vi "lab_3.vi"() -> ()   [LabVIEW 2016]
uses:
  <vilib>/myRIO/Instrument Drivers/Onboard Devices/Accelerometer/typedefs/Accelerometer Reference.ctl
  <vilib>/myRIO/Common/Instrument Driver Framework/Utilities/typedefs/myRIO Generic Hardware Reference.ctl
  <vilib>/myRIO/Common/Instrument Driver Framework/Utilities/typedefs/Hardware Version Enum.ctl
  <vilib>/myRIO/Common/Instrument Driver Framework/Utilities/typedefs/myRIO v1.0 Reference.ctl
  <vilib>/myRIO/Common/Instrument Driver Framework/Utilities/typedefs/Generic FPGA Reference.ctl
  <vilib>/myRIO/Common/Instrument Driver Framework/myRIO v1.0/Accelerometer/typedefs/Accelerometer Channels List.ctl
  <vilib>/myRIO/Common/Instrument Driver Framework/myRIO v1.0/Accelerometer/typedefs/Accelerometer Channels Enum.ctl
  <vilib>/userdefined/High Color/nirio_resource_hc.ctl
  <vilib>/myRIO/Instrument Drivers/Onboard IO/DIO/typedefs/DIO Reference.ctl
  <vilib>/myRIO/Common/Instrument Driver Framework/myRIO v1.0/DIO/typedefs/DIO Channels List.ctl
  <vilib>/myRIO/Common/Instrument Driver Framework/myRIO v1.0/DIO/typedefs/DIO Channels Enum.ctl
  <vilib>/myRIO/Common/Instrument Driver Framework/Utilities/vis/Is FPGA Ref Available.vi
  <vilib>/myRIO/Common/Instrument Driver Framework/myRIO v1.0/Accelerometer/vis/myRIO v1.1 Open Accelerometer.vi
  <vilib>/myRIO/Instrument Drivers/Onboard Devices/Accelerometer/vis/Read.vi
  <vilib>/myRIO/Common/Instrument Driver Framework/myRIO v1.0/DIO/vis/myRIO v1.1 Open DIO.vi
  <vilib>/myRIO/Instrument Drivers/Onboard IO/DIO/vis/Write.vi
  <vilib>/myRIO/Common/Instrument Driver Framework/Utilities/vis/Validate Channels.vi
  <vilib>/myRIO/Common/Instrument Driver Framework/myRIO v1.0/Accelerometer/vis/myRIO v1.0 Reserve Accelerometer.vi
  <vilib>/myRIO/Common/Instrument Driver Framework/myRIO v1.0/UART/vis/myRIO v1.0 Close UART.vi
  <vilib>/myRIO/Common/Instrument Driver Framework/myRIO v1.0/DIO/vis/myRIO v1.0 Reserve DIO.vi
  <vilib>/myRIO/Common/Instrument Driver Framework/myRIO v1.0/Resource Manager/vis/myRIO v1.0 Reserve Channel List.vi
  <vilib>/myRIO/Common/Instrument Driver Framework/myRIO v1.0/Accelerometer/vis/myRIO v1.0 Build MUX Configuration Accelerometer.vi
  <vilib>/myRIO/Common/Instrument Driver Framework/myRIO v1.0/DIO/vis/myRIO v1.0 Build MUX Configuration DIO.vi
  <vilib>/myRIO/Common/Instrument Driver Framework/myRIO v1.0/Resource Manager/vis/myRIO v1.0 Reserve Channel.vi
  <vilib>/myRIO/Common/Instrument Driver Framework/myRIO v1.0/Resource Manager/vis/myRIO v1.0 Unreserve Channel.vi
  <vilib>/myRIO/Common/Instrument Driver Framework/myRIO v1.0/Resource Manager/vis/myRIO v1.0 Create Configuration List.vi
  <vilib>/myRIO/Common/Instrument Driver Framework/myRIO v1.0/Resource Manager/vis/myRIO v1.0 Build Mutex Name.vi
  <vilib>/Utility/VariantDataType/GetNumericInfo.vi
  <vilib>/Utility/error.llb/Error Cluster From Error Code.vi
  <vilib>/myRIO/Common/Instrument Driver Framework/myRIO v1.0/myRIO v1.1 Open.vi
  <vilib>/myRIO/Common/Instrument Driver Framework/myRIO v1.0/Accelerometer/vis/myRIO v1.0 Get Scaling Constant Accelerometer.vi
  <vilib>/myRIO/Common/Instrument Driver Framework/Utilities/vis/IO Manager.vi
  <vilib>/myRIO/Common/Instrument Driver Framework/Utilities/vis/Configuration Manager.vi
  <vilib>/myRIO/Common/Instrument Driver Framework/myRIO v1.0/myRIO v1.0 Close.vi
  <vilib>/myRIO/Common/Instrument Driver Framework/myRIO v1.0/Accelerometer/vis/myRIO v1.0 Read Accelerometer.vi
  <vilib>/Analysis/Matrix/Numeric/Conversions/Matrix To Array - RM.vi
  <vilib>/myRIO/Common/Instrument Driver Framework/Utilities/vis/FPGA Ref Manager.vi
  <vilib>/myRIO/Common/Instrument Driver Framework/myRIO v1.0/myRIO v1.0 Reset FPGA.vi
  <vilib>/myRIO/Common/Instrument Driver Framework/myRIO v1.0/IRQ/vis/myRIO v1.0 IRQ Info FGV.vi
  <vilib>/myRIO/Common/Instrument Driver Framework/myRIO v1.0/IRQ/vis/myRIO v1.0 Timer IRQ Info FGV.vi
  <vilib>/myRIO/Common/Instrument Driver Framework/myRIO v1.0/IRQ/vis/myRIO v1.0 ISR Agent.vi
  <vilib>/myRIO/Common/Instrument Driver Framework/myRIO v1.0/Resource Manager/vis/myRIO v1.0 Configure IO.vi
  <vilib>/myRIO/Common/Instrument Driver Framework/myRIO v1.0/DIO/vis/myRIO v1.0 Write DIO.vi
  <vilib>/myRIO/Express VI/Onboard Devices/Accelerometer/Accelerometer Express VI.xnode
  <vilib>/myRIO/Instrument Drivers/Onboard Devices/Accelerometer/vis/myRIO Accelerometer Open.xnode
  <vilib>/myRIO/Express VI/Onboard Devices/LED/LED Express VI.xnode
  <vilib>/myRIO/Instrument Drivers/Onboard IO/DIO/vis/myRIO DIO Open.xnode
  <vilib>/myRIO/Instrument Drivers/Onboard Devices/Accelerometer/Accelerometer.lvlib
  <vilib>/myRIO/Instrument Drivers/Utilities/Utilities.lvlib
  <vilib>/Analysis/Matrix/NI_Matrix.lvlib
  <vilib>/myRIO/Instrument Drivers/Onboard IO/DIO/DIO.lvlib
panel:
  in  "ACTIVATION":bool
  in  "STOP INFERENCE":bool
  in  "WRITE WEIGHTS":bool=TRUE
  in  "WRITE DATA":bool
  in  "Weights Source":bool=TRUE
  in  "START INFERENCE":bool
  in  "BEGIN TRAINING MODE":bool
  in  "BEGIN INFERENCE MODE":bool
  in  "Mode Initialize":T1(ring)=enum."inference"
  in  "Validation Split":dbl=0.20000000000000015 min=0.0 max=1.0 step=0.1
  out "Loss":cluster{dbl, dbl}(graph)
  in  "Learning Rate":dbl=0.01 step=0.005
  out "Training Status":string
  in  "START TRAINING":bool
  out "Input Data":dbl[][](array[numeric])
  out "Total # of Samples":i32
  out "Targets":dbl[](array[numeric])
  in  "STOP TRAINING":bool
  in  "# ouputs":i32=3
  in  "# inputs":i32=5
  in  "# nodes per hidden layer":i32=8
  in  "# hidden layers":i32=1
  in  "Data Source":bool=TRUE
  out "Shuffled Targets":dbl[](array[numeric])
  out "Shuffled Input Data":dbl[][](array[numeric])
  in  "# of Samples to collect":i32
  in  "NEXT TARGET":bool
  out "Mode Status":string
  in  "Set Target (0, 1, 2)":i8 min=0 max=3
  out "# of Samples for current target":i32
  in  "Main Loop STOP":bool
  out "error out":errorcluster
  out "MyRIO Accelerometer":T2(graph)
  out "MyRIO Angular Position":cluster{dbl, dbl}(graph)
  in  "FILTER ON/OFF":bool=TRUE
  in  "Smoothing Factor":dbl(slide)=0.17171717171717182 min=-1.0 max=1.0 step=0.05 scale=-1.0..1.0
  # "Lab 4: Example Submission"
  # "Author: Adam Cavatassi, McGill University, 2018"
  # "Main Control"
  # "Training Control"
  # "ON - Shared Variable"
  # "OFF - Local Data"
  # "Inference Control"
  # "ON - Shared Variable"
  # "OFF - Local Data"
  # "ON - reLU"
  # "OFF - sigmoid Data"
  # "Data Generation Control"
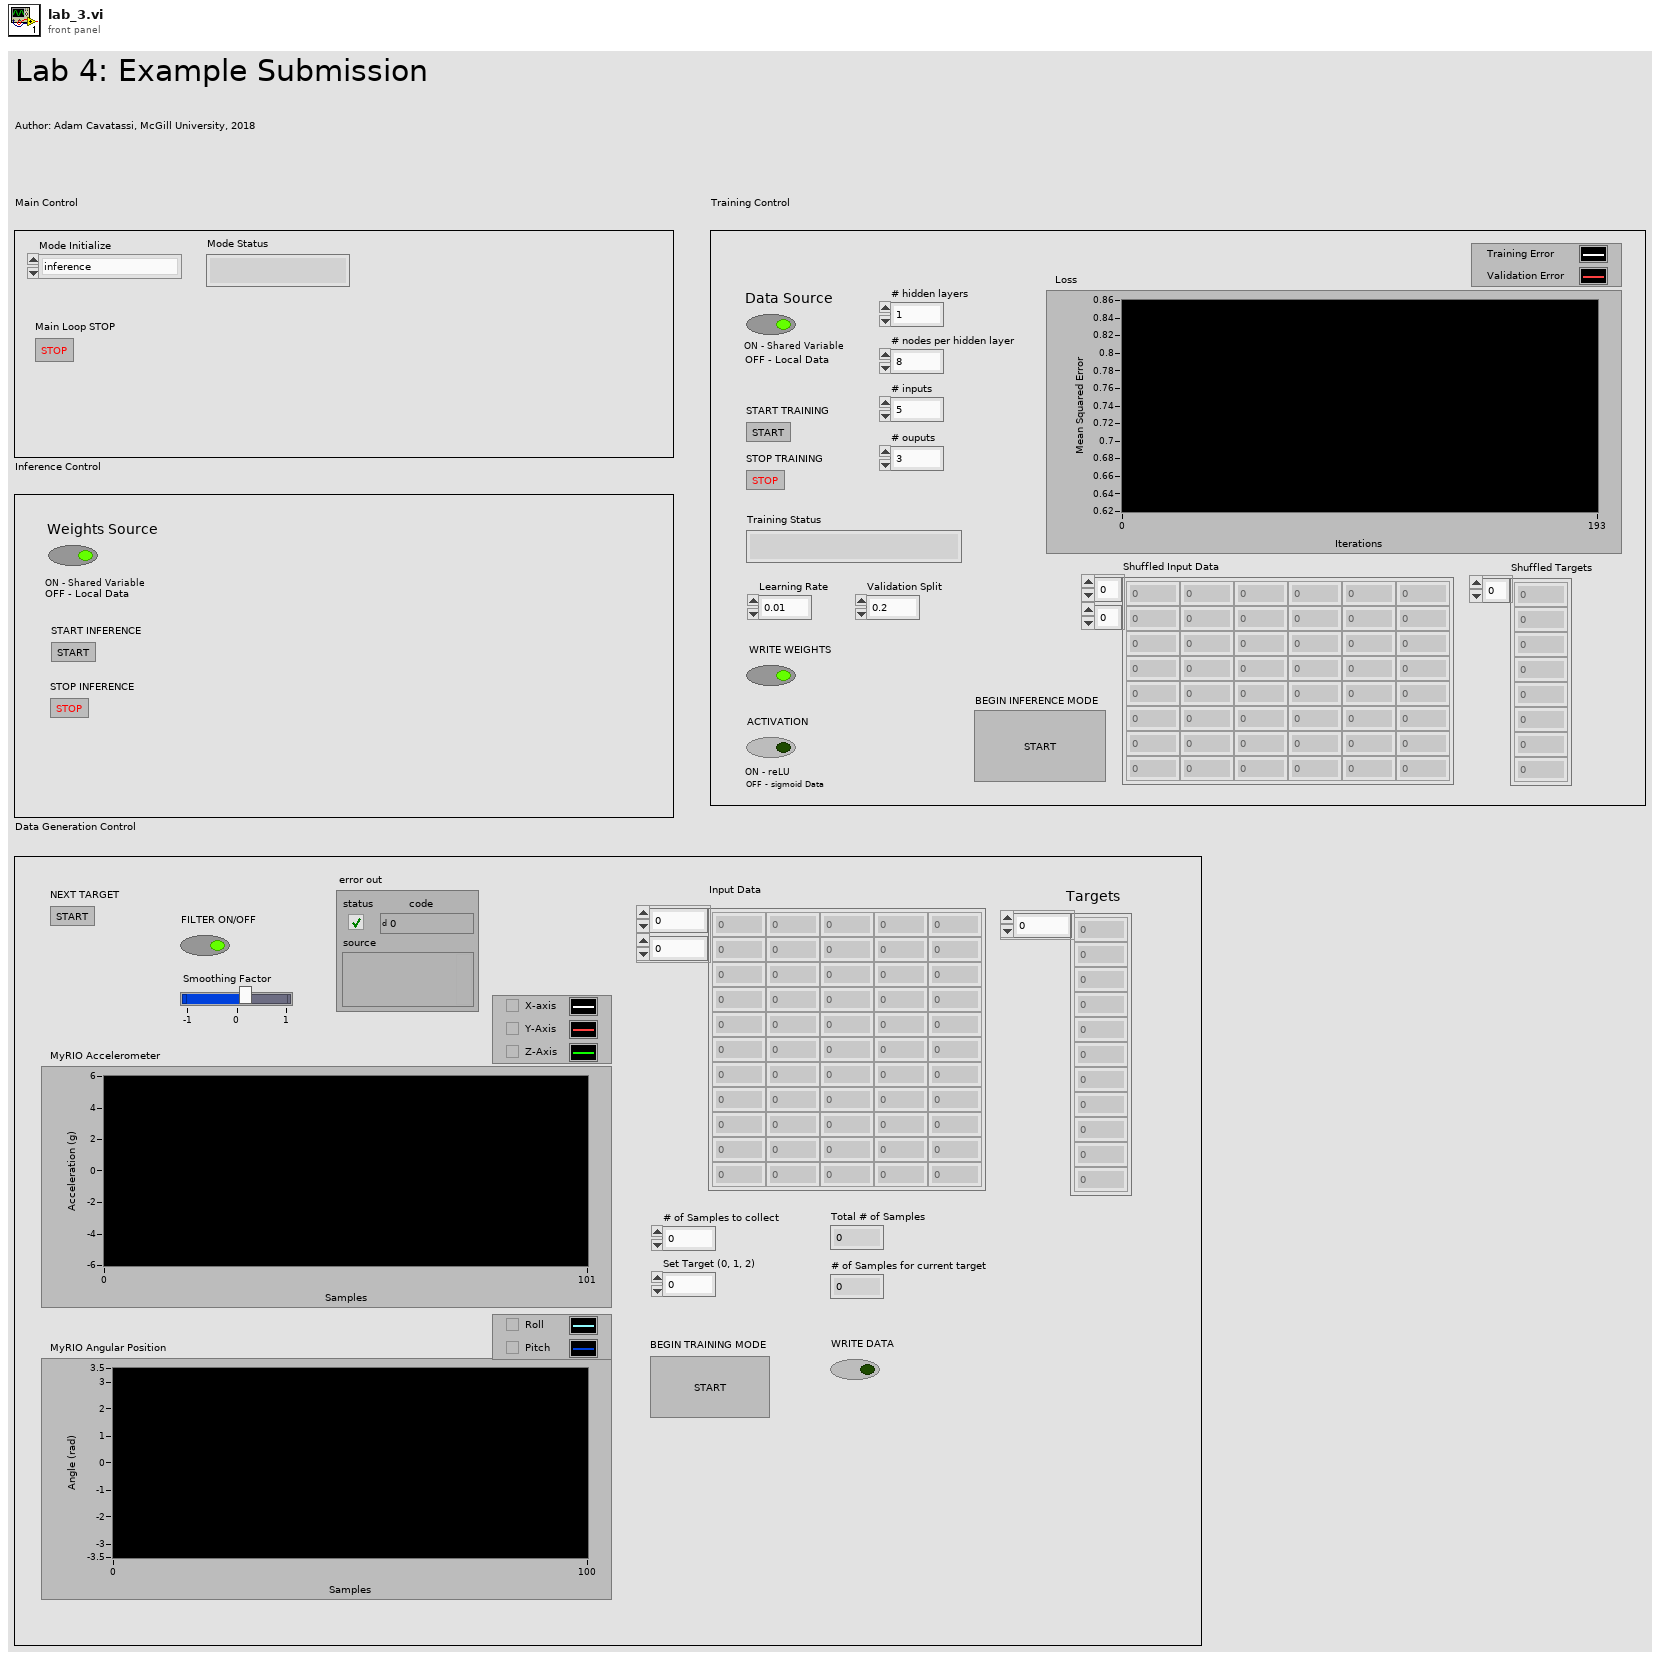
[diagram p1: front panel]
types:
  T1 = enum16{"data_collection", "network_train", "inference"}
  T2 = cluster{"X-Axis":dbl, "Y-Axis":dbl, "Z-Axis":dbl}
  T3 = typedef "Accelerometer.lvlib/Accelerometer Reference.ctl" = cluster{"myRIO Reference":T4, "Accelerometer Channels List":T8, "LSB Weight":dbl}
  T4 = typedef "myRIO Generic Hardware Reference.ctl" = cluster{"myRIO Model":T5, "myRIO Hardware Reference":T6}
  T5 = typedef "Hardware Version Enum.ctl" = enum16{"Unknown", "myRIO-1900", "myRIO-1950", "roboRIO", "NI ELVIS RIO CM"}
  T6 = typedef "myRIO v1.0 Reference.ctl" = cluster{"Generic FPGA Reference":T7, "Allow multiple opens":bool}
  T7 = typedef "Generic FPGA Reference.ctl" = refnum<k20>
  T8 = typedef "Accelerometer Channels List.ctl" = T9[]
  T9 = typedef "Accelerometer Channels Enum.ctl" = enum16{"Not Connected", "X-Axis", "Y-Axis", "Z-Axis"}
  T10 = typedef "nirio_resource_hc.ctl" = tag
  T11 = typedef "DIO.lvlib/DIO Reference.ctl" = cluster{"myRIO Reference":T4, "DIO Channels List":T12}
  T12 = typedef "DIO Channels List.ctl" = T13[]
  T13 = typedef "DIO Channels Enum.ctl" = enum16{"Not Connected", "C/DIO0", "C/DIO1", "C/DIO2", "C/DIO3", "C/DIO4", "C/DIO5", "C/DIO6", "C/DIO7", "A/DIO0", "A/DIO1", "A/DIO2", "A/DIO3", "A/DIO4", "A/DIO5", "A/DIO6", "A/DIO7", "A/DIO8", "A/DIO9", "A/DIO10", "A/DIO11", "A/DIO12", "A/DIO13", "A/DIO14", "A/DIO15", "B/DIO0", "B/DIO1", "B/DIO2", "B/DIO3", "B/DIO4", "B/DIO5", "B/DIO6", "B/DIO7", "B/DIO8", "B/DIO9", "B/DIO10", "B/DIO11", "B/DIO12", "B/DIO13", "B/DIO14", "B/DIO15", "LED0", "LED1", "LED2", "LED3", "Button0", "DIO/DIO0", "DIO/DIO1", "DIO/DIO2", "DIO/DIO3", "DIO/DIO4", "DIO/DIO5", "DIO/DIO6", "DIO/DIO7", "DIO/DIO8", "DIO/DIO9", "SPI/CS0", "SPI/CS1", "SPI/CS2", "SPI/CS3", "LED RADIO (Green)", "LED RADIO (Red)", "LED COMM (Green)", "LED COMM (Red)", "LED MODE (Green)", "LED MODE (Red)"}
  T14 = typedef "NI_Matrix.lvlib/RealMatrix.ctl" = dbl[][]
  T15 = cluster{"number: 0 to 1":dbl, dbl[], "Numeric":dbl}
  T16 = cluster{"number: 0 to 1":dbl, dbl[], "Numeric":dbl}[]
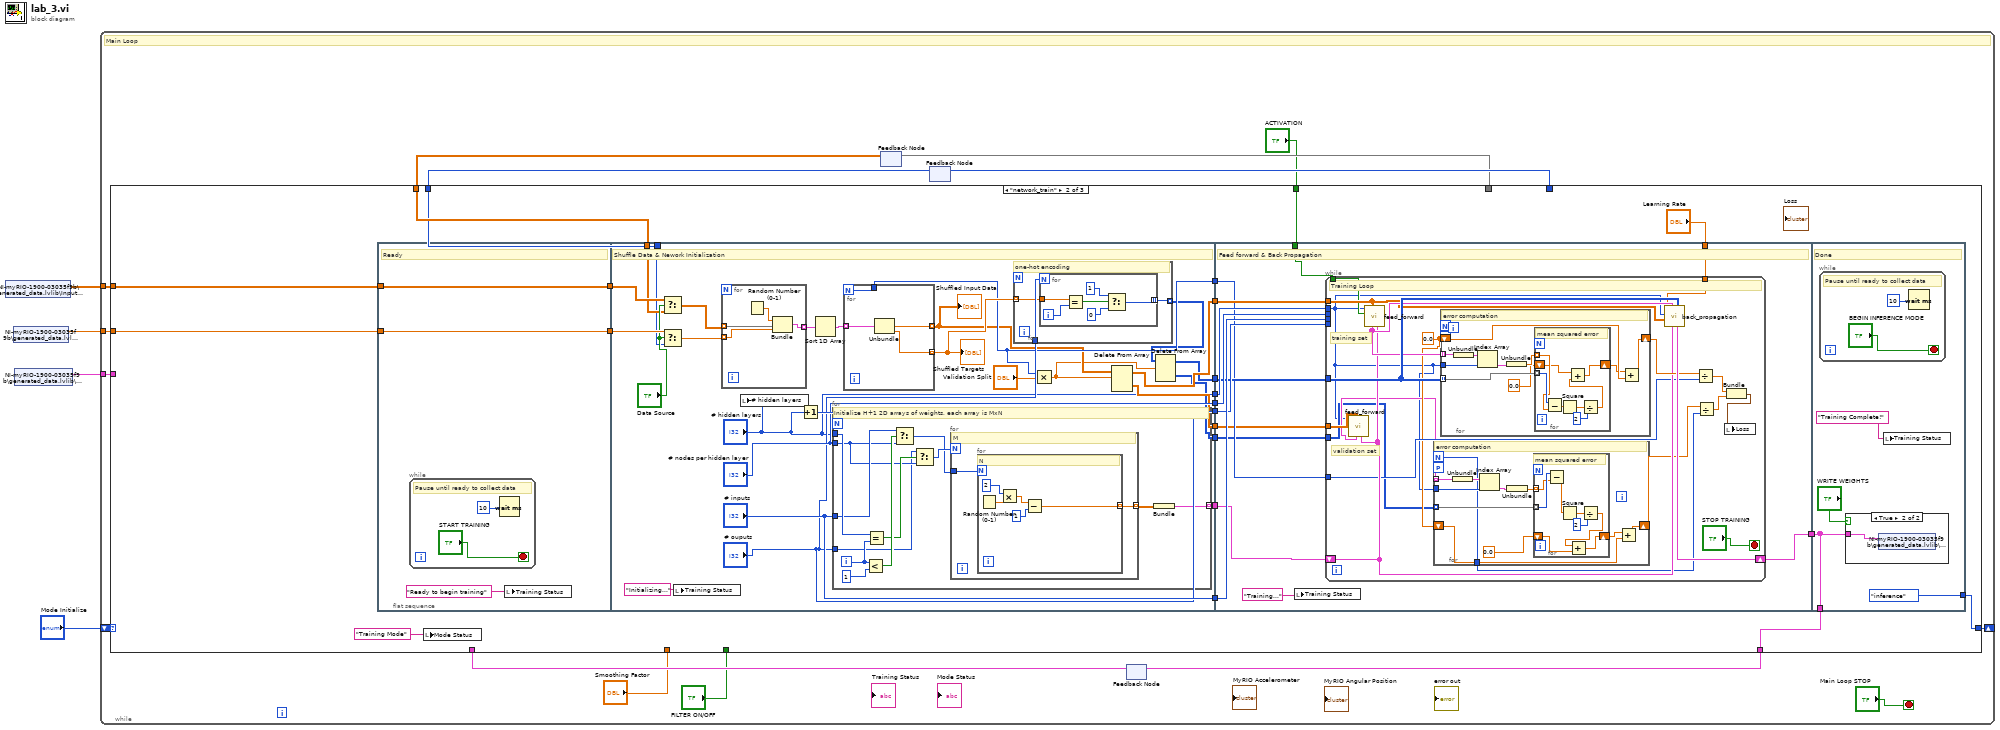
[diagram p0: block diagram]
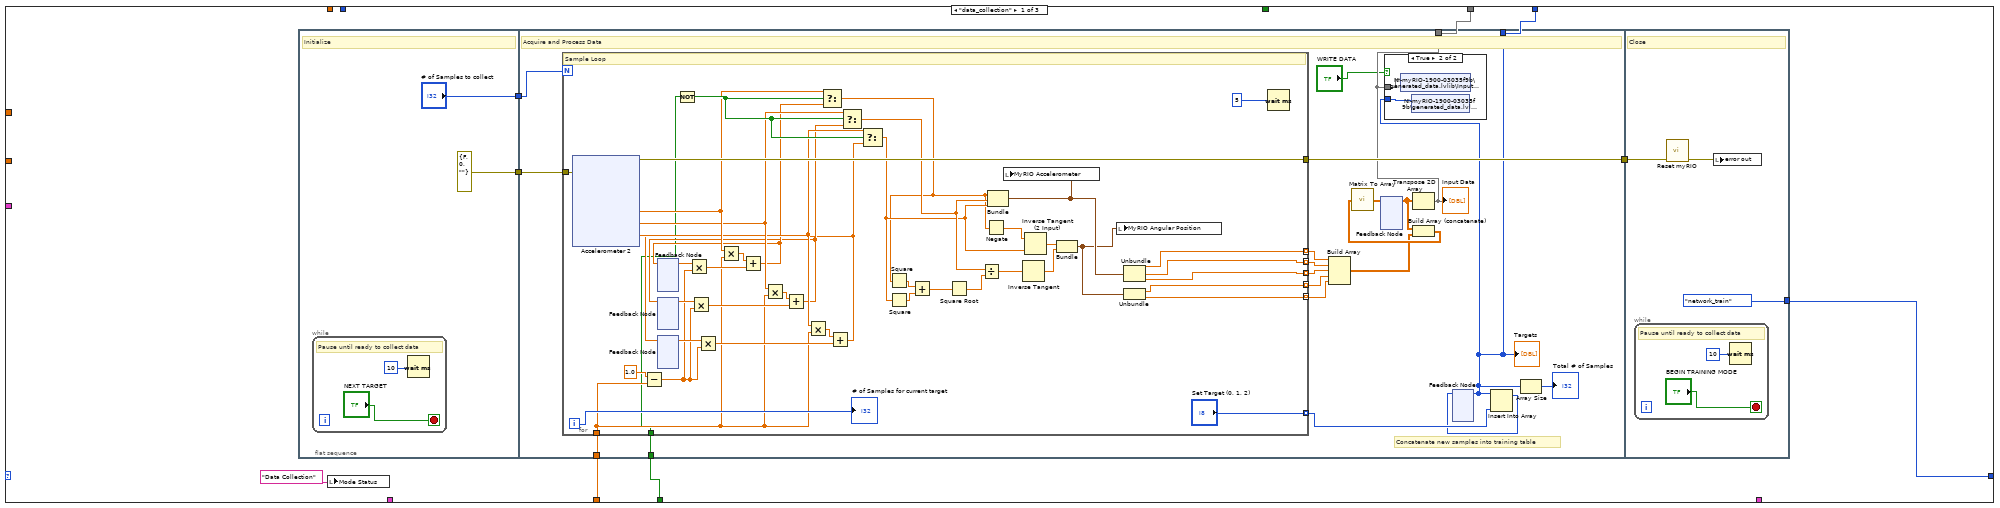
[diagram p2: hidden frame]
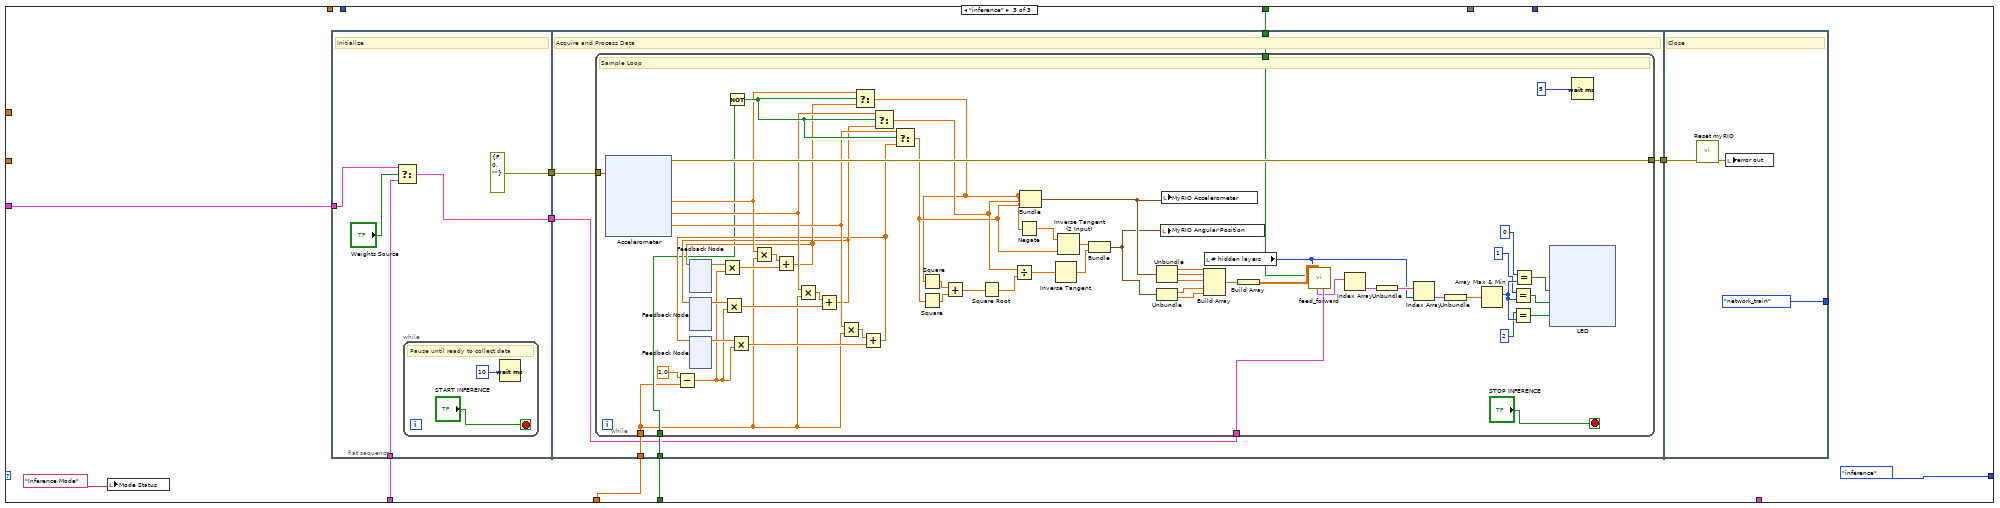
[diagram p5: hidden frame]
diagram:
  n1 = shared-variable "NI-myRIO-1900-03035f9b\\generated_data.lvlib\\Input Data"() -> (w3:dbl[][])  [unwired: 1 in, 1 out]
  n2 = shared-variable "NI-myRIO-1900-03035f9b\\generated_data.lvlib\\Targets"() -> (w4:dbl[])  [unwired: 1 in, 1 out]
  n3 = shared-variable "NI-myRIO-1900-03035f9b\\generated_data.lvlib\\Weights"() -> (w1:cluster{dbl[][]}[])  [unwired: 1 in, 1 out]
  n4 = while {
    shift-right: [w18] -> _
    shift-left: "Mode Initialize" -> [w19]
    tunnel: w3 -> [w17]
    tunnel: w4 -> [w16]
    tunnel: w1 -> [w10]
    stop <- "Main Loop STOP" stop-if-true
    # "Main Loop"
    n5 = feedback #1() -> (w12:dbl[][])  [unwired: 1 in]
    n6 = feedback #2() -> (w14:i8[])  [unwired: 1 in]
    n7 = feedback #3() -> (w8:cluster{dbl[][]}[])  [unwired: 1 in]
    n8 = case shown="\"network_train\"" w19 {
      tunnel: [w26 _ _] -> w13
      tunnel: [w25 _ _] -> w15
      tunnel: [w23 w147 T1."inference" ("NETWORK MODE")] -> w18
      tunnel: w17 -> [_ w163 _]
      tunnel: w16 -> [_ w162 _]
      tunnel: w12 -> [_ w161 _]
      tunnel: w14 -> [_ w160 _]
      tunnel: [_ w144 _] -> w9
      tunnel: w10 -> [_ _ w314]
      tunnel: w8 -> [_ _ w313]
      tunnel: "Smoothing Factor" -> [w21 _ w310]
      tunnel: "FILTER ON/OFF" -> [w20 _ w311]
      tunnel: "ACTIVATION" -> [_ w143 w309]
      frame "data_collection" {
        n9 = flat-sequence {
          tunnel: [errorcluster {"status"=FALSE, "code"=0, "source"=""} ("error in (no error)")] -> w28
          tunnel: ["# of Samples to collect"] -> w24
          tunnel: w28 -> [w52]
          tunnel: [w51] -> w27
          tunnel: [w37] -> w26
          tunnel: [w36] -> w25
          tunnel: w24 -> [w45]
          tunnel: w21 -> [w34]
          tunnel: w20 -> [w33]
          tunnel: w27 -> [w139]
          tunnel: [T1."network_train" ("NETWORK MODE")] -> w23
          frame #0 {
            # "Initialize"
            n10 = while {
              stop <- "NEXT TARGET" stop-if-true
              # "Pause until ready to collect data"
              n11 = Wait (ms)(milliseconds to wait=10) -> ()  [unwired: 1 out]
            }
          }
          frame #1 {
            # "Concatenate new samples into training table"
            # "Acquire and Process Data"
            n12 = for {
              N: w45 -> [_]
              tunnel: w52 -> [w96]
              tunnel: [w95] -> w51
              tunnel: [w66] -> w46 mode=indexing
              tunnel: [w65] -> w50 mode=indexing
              tunnel: [w64] -> w49 mode=indexing
              tunnel: [w63] -> w48 mode=indexing
              tunnel: [w62] -> w47 mode=indexing
              tunnel: ["Set Target (0, 1, 2)"] -> w43 mode=indexing
              tunnel: w34 -> [w58]
              tunnel: w33 -> [w57]
              i -> [w59]
              # "Sample Loop"
              n13 = xnode "Accelerometer 2"("error in (no error)"=w96) -> ("X-Axis"=w75:dbl, "Y-Axis"=w74:dbl, "Z-Axis"=w71:dbl, "error out"=w95:errorcluster)
              n14 = Subtract(x=1.0, y=w58) -> (x-y=w76:dbl)
              n15 = feedback #4() -> (w86:dbl)  [unwired: 1 in]
              n16 = feedback #5() -> (w85:dbl)  [unwired: 1 in]
              n17 = feedback #6() -> (w84:dbl)  [unwired: 1 in]
              n18 = Not(x=w57) -> (.not. x?=w80:bool)
              n19 = Multiply(x=w86, y=w76) -> (x*y=w79:dbl)
              n20 = Multiply(x=w85, y=w76) -> (x*y=w78:dbl)
              n21 = Multiply(x=w84, y=w76) -> (x*y=w77:dbl)
              n22 = Multiply(x=w75, y=w58) -> (x*y=w72:dbl)
              n23 = Add(x=w72, y=w79) -> (x+y=w69:dbl)
              n24 = feedback-in #4(w69) -> ()
              n25 = Multiply(x=w74, y=w58) -> (x*y=w73:dbl)
              n26 = Add(x=w73, y=w78) -> (x+y=w68:dbl)
              n27 = feedback-in #5(w68) -> ()
              n28 = Multiply(x=w71, y=w58) -> (x*y=w70:dbl)
              n29 = Select(t=w75, s=w80, f=w69) -> (s? t:f=w61:dbl)
              n30 = Add(x=w70, y=w77) -> (x+y=w67:dbl)
              n31 = feedback-in #6(w67) -> ()
              n32 = Select(t=w74, s=w80, f=w68) -> (s? t:f=w82:dbl)
              n33 = Select(t=w71, s=w80, f=w67) -> (s? t:f=w81:dbl)
              n34 = Square(x=w61) -> (x^2=w89:dbl)
              n35 = Square(x=w81) -> (x^2=w94:dbl)
              n36 = Add(x=w89, y=w94) -> (x+y=w93:dbl)
              n37 = Square Root(x=w93) -> (sqrt(x)=w92:dbl)
              n38 = Divide(x=w82, y=w92) -> (x/y=w91:dbl)
              n39 = Negate(x=w61) -> (-x=w88:dbl)
              n40 = Bundle("X-Axis"=w61, "Y-Axis"=w82, "Z-Axis"=w81) -> (w56:T2)  [unwired: 1 in]
              n41 = local write "MyRIO Accelerometer"(w56) -> ()
              n42 = Inverse Tangent(1:w91) -> (0:w90:dbl)
              n43 = Inverse Tangent (2 Input)(1:w81, 2:w88) -> (0:w87:dbl)
              n44 = Bundle(w87, w90) -> (w55:cluster{dbl, dbl})  [unwired: 1 in]
              n45 = local write "MyRIO Angular Position"(w55) -> ()
              n46 = Unbundle(w56) -> ("X-Axis"=w66:dbl, "Y-Axis"=w65:dbl, "Z-Axis"=w64:dbl)
              n47 = Unbundle(w55) -> (w63:dbl, w62:dbl)
              n48 = Wait (ms)(milliseconds to wait=5) -> ()  [unwired: 1 out]
              "# of Samples for current target" <- w59
            }
            n49 = Build Array(w46, w50, w49, w48, w47) -> (w38:dbl[][])
            n50 = feedback #7() -> (w39:dbl[][])  [unwired: 1 in]
            n51 = Transpose 2D Array(2D array=w39) -> (transposed array=w37:dbl[][])
            "Input Data" <- w37
            n52 = Build Array (concatenate)(w39, w38) -> (w40:T14)
            n53 = call-poly <vilib>:"Matrix To Array.vi"("Real Matrix"=w40) -> ("Real 2D Array"=w41:dbl[][])
            n54 = feedback-in #7(w41) -> ()
            n55 = feedback #8() -> (w36:i8[])  [unwired: 1 in]
            "Targets" <- w36
            n56 = case shown="True" "WRITE DATA" {
              tunnel: w37 -> [_ w54]
              tunnel: w36 -> [_ w53]
              frame False {
              }
              frame True {
                n57 = shared-variable "NI-myRIO-1900-03035f9b\\generated_data.lvlib\\Input Data"(w54) -> ()  [unwired: 1 in, 1 out]
                n58 = shared-variable "NI-myRIO-1900-03035f9b\\generated_data.lvlib\\Targets"(w53) -> ()  [unwired: 1 in, 1 out]
              }
            }
            n59 = Insert Into Array(array=w36, new element=w43) -> (w42:i8[])  [unwired: 1 in]
            n60 = feedback-in #8(w42) -> ()
            n61 = Array Size(array=w36) -> (size(s)=→"Total # of Samples":i32)
          }
          frame #2 {
            # "Close"
            n62 = while {
              stop <- "BEGIN TRAINING MODE" stop-if-true
              # "Pause until ready to collect data"
              n63 = Wait (ms)(milliseconds to wait=10) -> ()  [unwired: 1 out]
            }
            n64 = call <vilib>:"Reset myRIO.vi"("error in (no error)"=w139) -> ("error out"=w137:errorcluster)  [unwired: 10 in]
            n65 = local write "error out"(w137) -> ()
          }
        }
        n66 = local write "Mode Status"("Data Collection") -> ()
      }
      frame "network_train" {
        n67 = flat-sequence {
          tunnel: w162 -> [w165]
          tunnel: w163 -> [w166]
          tunnel: [w166] -> w153
          tunnel: [w165] -> w152
          tunnel: w161 -> [w187]
          tunnel: w160 -> [w186]
          tunnel: [w182] -> w159
          tunnel: [w172] -> w158
          tunnel: ["# hidden layers"] -> w157
          tunnel: ["# nodes per hidden layer"] -> w156
          tunnel: ["# inputs"] -> w155
          tunnel: ["# ouputs"] -> w154
          tunnel: w153 -> [w192]
          tunnel: w152 -> [w190]
          tunnel: [w171] -> w151
          tunnel: [w177] -> w150
          tunnel: [w173] -> w149
          tunnel: [w170] -> w148
          tunnel: w159 -> [w238]
          tunnel: w158 -> [w244]
          tunnel: w157 -> [w243]
          tunnel: w156 -> [w242]
          tunnel: w155 -> [w241]
          tunnel: w154 -> [w240]
          tunnel: w151 -> [w237]
          tunnel: w150 -> [w236]
          tunnel: w149 -> [w235]
          tunnel: w148 -> [w234]
          tunnel: [w233] -> w145
          tunnel: w143 -> [w232]
          tunnel: "Learning Rate" -> [w231]
          tunnel: [T1."inference" ("NETWORK MODE")] -> w147
          tunnel: w145 -> [w304]
          tunnel: [w304] -> w144
          frame #0 {
            # "Ready"
            n68 = while {
              stop <- "START TRAINING" stop-if-true
              # "Pause until ready to collect data"
              n69 = Wait (ms)(milliseconds to wait=10) -> ()  [unwired: 1 out]
            }
            n70 = local write "Training Status"("Ready to begin training") -> ()
          }
          frame #1 {
            # "Shuffle Data & Nework Initialization"
            n71 = Select(t=w192, s="Data Source", f=w187) -> (s? t:f=w191:dbl[][])
            n72 = Select(t=w190, s="Data Source", f=w186) -> (s? t:f=w189:dbl[])
            n73 = local write "Training Status"("Initializing...") -> ()
            n74 = for {
              tunnel: w191 -> [w228] mode=indexing
              tunnel: w189 -> [w230] mode=indexing
              tunnel: [w227] -> w194 mode=indexing
              n75 = Random Number (0-1)() -> (number: 0 to 1=w229:dbl)
              n76 = Bundle("number: 0 to 1"=w229, w228, "Numeric"=w230) -> (w227:T15)  [unwired: 1 in]
            }
            n77 = local write "# hidden layers"("# hidden layers") -> ()
            n78 = Increment(x="# hidden layers") -> (x+1=w185:i32)
            n79 = Sort 1D Array(array=w194) -> (sorted array=w193:T16)
            n80 = for {
              N: w185 -> [_]
              tunnel: "# hidden layers" -> [w215]
              tunnel: "# inputs" -> [w214]
              tunnel: "# nodes per hidden layer" -> [w208]
              tunnel: "# ouputs" -> [w207]
              tunnel: [w204] -> w182 mode=indexing
              i -> [w209]
              # "Initialize H+1 2D arrays of weights, each array is MxN"
              n81 = Less?(x=w209, y=1) -> (x < y?=w213:bool)
              n82 = Equal?(x=w215, y=w209) -> (x = y?=w212:bool)
              n83 = Select(t=w214, s=w213, f=w208) -> (s? t:f=w206:i32)
              n84 = Select(t=w207, s=w212, f=w208) -> (s? t:f=w211:i32)
              n85 = for {
                N: w211 -> [_]
                tunnel: [w217] -> w205 mode=indexing
                tunnel: w206 -> [w216]
                # "M"
                n86 = for {
                  N: w216 -> [_]
                  tunnel: [w218] -> w217 mode=indexing
                  # "N"
                  n87 = Random Number (0-1)() -> (number: 0 to 1=w222:dbl)
                  n88 = Multiply(x=2, y=w222) -> (x*y=w220:dbl)
                  n89 = Subtract(x=w220, y=1) -> (x-y=w218:dbl)
                }
              }
              n90 = Bundle(w205) -> (w204:cluster{dbl[][]})  [unwired: 1 in]
            }
            n91 = for {
              N -> [w223]
              tunnel: w193 -> [w225] mode=indexing
              tunnel: [w226] -> w176 mode=indexing
              tunnel: [w224] -> w179 mode=indexing
              tunnel: [w223] -> w177
              n92 = Unbundle(w225) -> (w226:dbl[], "Numeric"=w224:dbl)  [unwired: 1 out]
            }
            "Shuffled Input Data" <- w176
            "Shuffled Targets" <- w179
            n93 = for {
              tunnel: "# ouputs" -> [w197]
              tunnel: w179 -> [w196] mode=indexing
              tunnel: [w195] -> w175 mode=indexing
              # "one-hot encoding"
              n94 = for {
                N: w197 -> [_]
                tunnel: w196 -> [w202]
                tunnel: [w198] -> w195 mode=indexing
                i -> [w203]
                n95 = Equal?(x=w202, y=w203) -> (x = y?=w201:bool)
                n96 = Select(t=1, s=w201, f=0) -> (s? t:f=w198:i32)
              }
            }
            n97 = Multiply(x=w177, y="Validation Split") -> (x*y=w174:dbl)
            n98 = Delete From Array(array=w176, length=w174) -> (deleted portion=w173:dbl[][], array with subset deleted=w172:dbl[][])  [unwired: 2 in]
            n99 = Delete From Array(array=w175, length=w174) -> (deleted portion=w170:i32[][], array with subset deleted=w171:i32[][])  [unwired: 2 in]
          }
          frame #2 {
            # "Feed forward & Back Propagation"
            n100 = local write "Training Status"("Training...") -> ()
            n101 = while {
              tunnel: w244 -> [w261]
              tunnel: w243 -> [w248]
              tunnel: w242 -> [_]
              tunnel: w241 -> [_]
              tunnel: w240 -> [_]
              shift-right: [w262] -> w233
              shift-left: w238 -> [w259]
              tunnel: w237 -> [w264]
              tunnel: w236 -> [w255]
              tunnel: w235 -> [w258]
              tunnel: w234 -> [w251]
              tunnel: w232 -> [w249]
              tunnel: w231 -> [w247]
              stop <- "STOP TRAINING" stop-if-true
              w253 = 0.0
              # "training set"
              # "validation set"
              # "Training Loop"
              n102 = call "feed_forward.vi"("Weights Cluster"=w259, "Input Data"=w258, "# hidden layers"=w248) -> ("Neurons"=w252:cluster{"Array":cluster{"Array 2":dbl[]}[]}[])  [unwired: 8 in]
              n103 = call "feed_forward.vi"("Weights Cluster"=w259, "Input Data"=w261, "act"=w249, "# hidden layers"=w248) -> ("Neurons"=w263:cluster{"Array":cluster{"Array 2":dbl[]}[]}[])  [unwired: 7 in]
              n104 = for {
                N -> [w265]
                tunnel: w248 -> [w273]
                tunnel: w252 -> [w275] mode=indexing
                shift-right: [w267] -> w254
                shift-left: w253 -> [w266]
                tunnel: w251 -> [w271] mode=indexing
                tunnel: [w265] -> w250
                workers-P: _ -> [_]
                # "error computation"
                n105 = Unbundle(w275) -> ("Array"=w274:cluster{"Array 2":dbl[]}[])
                n106 = Index Array(array=w274, index=w273) -> (element=w272:cluster{"Array 2":dbl[]})
                n107 = Unbundle(w272) -> ("Array 2"=w270:dbl[])
                n108 = for {
                  tunnel: w271 -> [w280] mode=indexing
                  tunnel: w270 -> [w276] mode=indexing
                  shift-right: [w278] -> w268
                  shift-left: 0.0 -> [w279]
                  # "mean squared error"
                  n109 = Subtract(x=w280, y=w276) -> (x-y=w283:dbl)
                  n110 = Square(x=w283) -> (x^2=w282:dbl)
                  n111 = Divide(x=w282, y=2) -> (x/y=w277:dbl)
                  n112 = Add(x=w277, y=w279) -> (x+y=w278:dbl)
                }
                n113 = Add(x=w268, y=w266) -> (x+y=w267:dbl)
              }
              n114 = for {
                tunnel: w264 -> [w293] mode=indexing
                tunnel: w263 -> [w292] mode=indexing
                tunnel: w248 -> [w285]
                shift-right: [w286] -> w260
                shift-left: w253 -> [w288]
                workers-P: _ -> [_]
                # "error computation"
                n115 = Unbundle(w292) -> ("Array"=w291:cluster{"Array 2":dbl[]}[])
                n116 = Index Array(array=w291, index=w285) -> (element=w290:cluster{"Array 2":dbl[]})
                n117 = Unbundle(w290) -> ("Array 2"=w289:dbl[])
                n118 = for {
                  tunnel: w293 -> [w301] mode=indexing
                  tunnel: w289 -> [w297] mode=indexing
                  shift-right: [w294] -> w287
                  shift-left: 0.0 -> [w295]
                  # "mean squared error"
                  n119 = Subtract(x=w301, y=w297) -> (x-y=w300:dbl)
                  n120 = Square(x=w300) -> (x^2=w299:dbl)
                  n121 = Divide(x=w299, y=2) -> (x/y=w296:dbl)
                  n122 = Add(x=w295, y=w296) -> (x+y=w294:dbl)
                }
                n123 = Add(x=w287, y=w288) -> (x+y=w286:dbl)
              }
              n124 = call "back_propagation.vi"("Targets"=w264, "Old Weights"=w259, "Neurons"=w263, "Input Data"=w261, "# hidden layers"=w248, "Learning rate"=w247) -> ("New Weights"=w262:cluster{"Array":dbl[][]}[])  [unwired: 5 in]
              n125 = Divide(x=w260, y=w255) -> (x/y=w257:dbl)
              n126 = Divide(x=w254, y=w250) -> (x/y=w256:dbl)
              n127 = Bundle(w257, w256) -> (w246:cluster{dbl, dbl})  [unwired: 1 in]
              n128 = local write "Loss"(w246) -> ()
            }
          }
          frame #3 {
            # "Done"
            n129 = while {
              stop <- "BEGIN INFERENCE MODE" stop-if-true
              # "Pause until ready to collect data"
              n130 = Wait (ms)(milliseconds to wait=10) -> ()  [unwired: 1 out]
            }
            n131 = case shown="True" "WRITE WEIGHTS" {
              tunnel: w304 -> [_ w306]
              frame False {
              }
              frame True {
                n132 = shared-variable "NI-myRIO-1900-03035f9b\\generated_data.lvlib\\Weights"(w306) -> ()  [unwired: 1 in, 1 out]
              }
            }
            n133 = local write "Training Status"("Training Complete!") -> ()
          }
        }
        n134 = local write "Mode Status"("Training Mode") -> ()
      }
      frame "inference" {
        n135 = local write "Mode Status"("Inference Mode") -> ()
        n136 = flat-sequence {
          tunnel: [errorcluster {"status"=FALSE, "code"=0, "source"=""} ("error in (no error)")] -> w316
          tunnel: w314 -> [w321]
          tunnel: w313 -> [w320]
          tunnel: [w319] -> w312
          tunnel: w316 -> [w331]
          tunnel: [w330] -> w315
          tunnel: w312 -> [w327]
          tunnel: w311 -> [w329]
          tunnel: w310 -> [w328]
          tunnel: w309 -> [w326]
          tunnel: w315 -> [w469]
          tunnel: [T1."network_train" ("NETWORK MODE")] -> _
          frame #0 {
            # "Initialize"
            n137 = Select(t=w321, s="Weights Source", f=w320) -> (s? t:f=w319:cluster{dbl[][]}[])
            n138 = while {
              stop <- "START INFERENCE" stop-if-true
              # "Pause until ready to collect data"
              n139 = Wait (ms)(milliseconds to wait=10) -> ()  [unwired: 1 out]
            }
          }
          frame #1 {
            # "Acquire and Process Data"
            n140 = while {
              tunnel: w331 -> [w389]
              tunnel: [w388] -> w330
              tunnel: w329 -> [w357]
              tunnel: w328 -> [w356]
              tunnel: w327 -> [w355]
              tunnel: w326 -> [w340]
              stop <- "STOP INFERENCE" stop-if-true
              # "Sample Loop"
              n141 = xnode "Accelerometer"("error in (no error)"=w389) -> ("X-Axis"=w368:dbl, "Y-Axis"=w367:dbl, "Z-Axis"=w364:dbl, "error out"=w388:errorcluster)
              n142 = Subtract(x=1.0, y=w356) -> (x-y=w369:dbl)
              n143 = feedback #9() -> (w379:dbl)  [unwired: 1 in]
              n144 = feedback #10() -> (w378:dbl)  [unwired: 1 in]
              n145 = feedback #11() -> (w377:dbl)  [unwired: 1 in]
              n146 = Multiply(x=w379, y=w369) -> (x*y=w372:dbl)
              n147 = Multiply(x=w378, y=w369) -> (x*y=w371:dbl)
              n148 = Not(x=w357) -> (.not. x?=w373:bool)
              n149 = Multiply(x=w377, y=w369) -> (x*y=w370:dbl)
              n150 = Multiply(x=w368, y=w356) -> (x*y=w365:dbl)
              n151 = Add(x=w365, y=w372) -> (x+y=w362:dbl)
              n152 = feedback-in #9(w362) -> ()
              n153 = Multiply(x=w367, y=w356) -> (x*y=w366:dbl)
              n154 = Add(x=w366, y=w371) -> (x+y=w361:dbl)
              n155 = feedback-in #10(w361) -> ()
              n156 = Multiply(x=w364, y=w356) -> (x*y=w363:dbl)
              n157 = Select(t=w368, s=w373, f=w362) -> (s? t:f=w359:dbl)
              n158 = Add(x=w363, y=w370) -> (x+y=w360:dbl)
              n159 = feedback-in #11(w360) -> ()
              n160 = Select(t=w367, s=w373, f=w361) -> (s? t:f=w375:dbl)
              n161 = Select(t=w364, s=w373, f=w360) -> (s? t:f=w374:dbl)
              n162 = Square(x=w359) -> (x^2=w382:dbl)
              n163 = Square(x=w374) -> (x^2=w387:dbl)
              n164 = Add(x=w382, y=w387) -> (x+y=w386:dbl)
              n165 = Square Root(x=w386) -> (sqrt(x)=w385:dbl)
              n166 = Divide(x=w375, y=w385) -> (x/y=w384:dbl)
              n167 = Negate(x=w359) -> (-x=w381:dbl)
              n168 = Bundle("X-Axis"=w359, "Y-Axis"=w375, "Z-Axis"=w374) -> (w354:T2)  [unwired: 1 in]
              n169 = Inverse Tangent(1:w384) -> (0:w383:dbl)
              n170 = Inverse Tangent (2 Input)(1:w374, 2:w381) -> (0:w380:dbl)
              n171 = Bundle(w380, w383) -> (w353:cluster{dbl, dbl})  [unwired: 1 in]
              n172 = Unbundle(w354) -> ("X-Axis"=w352:dbl, "Y-Axis"=w351:dbl, "Z-Axis"=w350:dbl)
              n173 = Unbundle(w353) -> (w349:dbl, w348:dbl)
              n174 = local write "MyRIO Angular Position"(w353) -> ()
              n175 = local write "MyRIO Accelerometer"(w354) -> ()
              n176 = Build Array(w352, w351, w350, w349, w348) -> (w347:dbl[])
              n177 = local read "# hidden layers"() -> (w342:i32)
              n178 = Build Array(w347) -> (w346:dbl[][])
              n179 = call "feed_forward.vi"("Weights Cluster"=w355, "Input Data"=w346, "act"=w340, "# hidden layers"=w342) -> ("Neurons"=w345:cluster{"Array":cluster{"Array 2":dbl[]}[]}[])  [unwired: 7 in]
              n180 = Index Array(array=w345) -> (element=w344:cluster{"Array":cluster{"Array 2":dbl[]}[]})  [unwired: 1 in]
              n181 = Unbundle(w344) -> ("Array"=w343:cluster{"Array 2":dbl[]}[])
              n182 = Index Array(array=w343, index=w342) -> (element=w341:cluster{"Array 2":dbl[]})
              n183 = Unbundle(w341) -> ("Array 2"=w339:dbl[])
              n184 = Array Max & Min(array=w339) -> (max index (indices)=w335:i32)  [unwired: 3 out]
              n185 = Equal?(x=1, y=w335) -> (x = y?=w337:bool)
              n186 = Equal?(x=2, y=w335) -> (x = y?=w336:bool)
              n187 = Equal?(x=0, y=w335) -> (x = y?=w338:bool)
              n188 = xnode "LED"("pos0"=w338, "pos1"=w337, "pos2"=w336) -> ()  [unwired: 1 in, 1 out]
              n189 = Wait (ms)(milliseconds to wait=5) -> ()  [unwired: 1 out]
            }
          }
          frame #2 {
            # "Close"
            n190 = call <vilib>:"Reset myRIO.vi"("error in (no error)"=w469) -> ("error out"=w467:errorcluster)  [unwired: 10 in]
            n191 = local write "error out"(w467) -> ()
          }
        }
      }
    }
    n192 = feedback-in #1(w13) -> ()
    n193 = feedback-in #2(w15) -> ()
    n194 = feedback-in #3(w9) -> ()
  }
